vi "CurrentVIFolder.vi"(8 "error in (no error)":errorcluster caption="entrée d'erreur", 10 "Source":T1(ring), 11 "NomFichier":string) -> (0 "error out":errorcluster caption="sortie d'erreur", 2 "NomDuVI":string, 3 "Chemin":path)   [LabVIEW 2019]
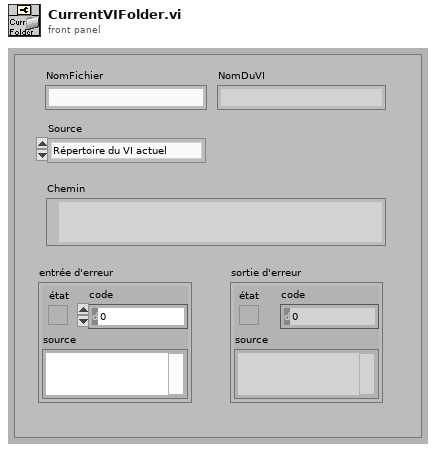
[diagram p1: front panel]
types:
  T1 = enum16{"Répertoire du VI actuel", "Répertoire du parent 1", "Répertoire du parent 2", "Répertoire du parent 3"}
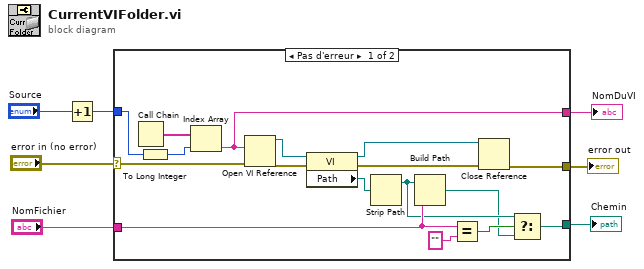
[diagram p0: block diagram]
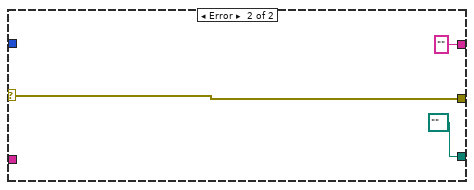
[diagram p2: hidden frame]
diagram:
  n1 = Increment(x="Source") -> (x+1=w2:T1)
  n2 = case shown="Pas d'erreur" "error in (no error)" {
    selector: "error in (no error)" -> [w21 w27]
    tunnel: [w19 w27] -> w6
    tunnel: "NomFichier" -> [w16 _]
    tunnel: [w11 path "" ("appended path")] -> w4
    tunnel: w2 -> [w10 _]
    tunnel: [w8 ""] -> w1
    frame No Error {
      n3 = Call Chain() -> (call chain=w24:string[])
      n4 = To Long Integer(number=w10) -> (32bit integer=w9:i32)
      n5 = Index Array(array=w24, index=w9) -> (element=w8:string)
      n6 = Open VI Reference(vi path=w8, error in (no error)=w21) -> (vi reference=w23:refnum<vi>, error out=w22:errorcluster)  [unwired: 4 in]
      n7 = property class="VI"(reference=w23, error in=w22) -> (reference out=w17:refnum<vi>, error out=w18:errorcluster, "Path"=w20:path)
      n8 = Strip Path(path=w20) -> (stripped path=w13:path)  [unwired: 1 out]
      n9 = Build Path(base path=w13, name or relative path=w16) -> (appended path=w12:path)
      n10 = Equal?(x=w16, y="") -> (x = y?=w14:bool)
      n11 = Close Reference(reference=w17, error in (no error)=w18) -> (error out=w19:errorcluster)
      n12 = Select(t=w13, s=w14, f=w12) -> (s? t:f=w11:path)
    }
    frame Error {
    }
  }
  "error out" <- w6
  "Chemin" <- w4
  "NomDuVI" <- w1
